vi "Read_calib_file.vi"(11 "string":string) -> (2 "output cluster":T1, 4 "Output Layer":cluster{"Array":dbl[][], "Array":dbl[][]}, 5 "Input Layer":cluster{"Array":dbl[][], "Array":dbl[][]}, 6 "Layer 2":cluster{"Array":dbl[][], "Array":dbl[][]}, 7 "Layer 1":cluster{"Array":dbl[][], "Array":dbl[][]})   [LabVIEW 2016]
uses:
  <vilib>/Utility/config.llb/Read Key (String).vi
  <vilib>/Utility/config.llb/NI_LVConfig.lvlib
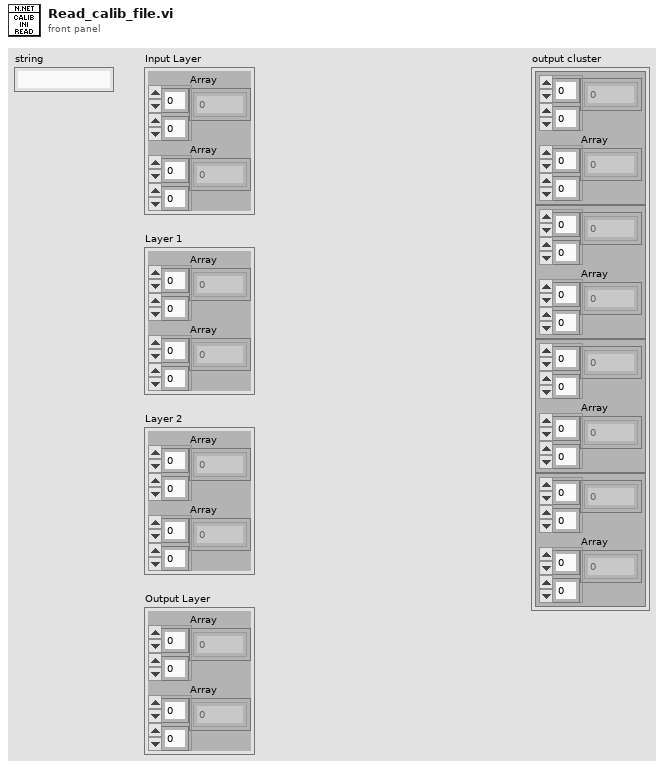
[diagram p1: front panel]
types:
  T1 = cluster{cluster{dbl[][], "Array":dbl[][]}, cluster{dbl[][], "Array":dbl[][]}, cluster{dbl[][], "Array":dbl[][]}, cluster{dbl[][], "Array":dbl[][]}}
  T2 = typedef "NI_LVConfig.lvlib/Config Data RefNum.ctl" = refnum<k1>
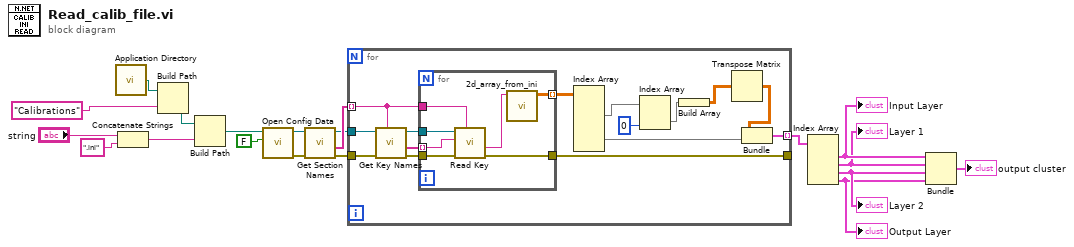
[diagram p0: block diagram]
diagram:
  n1 = call <vilib>:"Application Directory.vi"() -> ("Application Directory"=w6:path)
  n2 = Concatenate Strings("string", ".ini") -> (w18:string)
  n3 = Build Path(base path=w6, name or relative path="Calibrations" ("string")) -> (appended path=w8:path)
  n4 = Build Path(base path=w8, name or relative path=w18) -> (appended path=w19:path)
  n5 = call <vilib>:"Open Config Data.vi"("create file if necessary (T)"=FALSE, "configuration file path"=w19) -> ("error out"=w12:errorcluster, "refnum"=w11:T2)  [unwired: 7 in, 1 out]
  n6 = call <vilib>:"Get Section Names.vi"("error in (no error)"=w12, "refnum"=w11) -> ("error out"=w13:errorcluster, "section names"=w14:string[], "refnum out"=w9:T2)  [unwired: 7 in]
  n7 = for {
    tunnel: w13 -> [w34]
    tunnel: w14 -> [w33] mode=indexing
    tunnel: [w30] -> _
    tunnel: [w27] -> w15 mode=indexing
    tunnel: w9 -> [w25]
    n8 = call <vilib>:"Get Key Names.vi"("section"=w33, "error in (no error)"=w34, "refnum"=w25) -> ("error out"=w31:errorcluster, "key names"=w32:string[], "refnum out"=w26:T2)  [unwired: 5 in, 1 out]
    n9 = for {
      tunnel: w33 -> [w41]
      tunnel: w32 -> [w40] mode=indexing
      tunnel: w31 -> [w39]
      tunnel: [w38] -> w30
      tunnel: [w36] -> w29 mode=indexing
      tunnel: w26 -> [w35]
      n10 = call-poly <vilib>:"Read Key.vi"("section"=w41, "error in (no error)"=w39, "key"=w40, "refnum"=w35) -> ("error out"=w38:errorcluster, "value"=w37:string)  [unwired: 4 in, 2 out]
      n11 = call "2d_array_from_ini.vi"("Ini gene W"=w37) -> ("Array"=w36:dbl[][])  [unwired: 10 in]
    }
    n12 = Index Array(array=w29) -> (element #1=w24:dbl[][], element #2=w28:dbl[][])  [unwired: 6 in]
    n13 = Index Array(array=w24, index (col)=0 ("disabled index (col)")) -> (element=w22:dbl[])  [unwired: 1 in]
    n14 = Build Array(w22) -> (w21:dbl[][])
    n15 = Transpose Matrix(1:w21) -> (0:w20:dbl[][])
    n16 = Bundle(w20, "Array"=w28) -> (w27:cluster{dbl[][], "Array":dbl[][]})  [unwired: 1 in]
  }
  n17 = Index Array(array=w15) -> (element #1=w5:cluster{dbl[][], "Array":dbl[][]}, element #2=w4:cluster{dbl[][], "Array":dbl[][]}, element #3=w3:cluster{dbl[][], "Array":dbl[][]}, element #4=w2:cluster{dbl[][], "Array":dbl[][]})  [unwired: 4 in]
  "Output Layer" <- w2
  "Layer 2" <- w3
  "Layer 1" <- w4
  "Input Layer" <- w5
  n18 = Bundle(w5, w4, w3, w2) -> (→"output cluster":T1)  [unwired: 1 in]
